vi "Init.vi"(8 "error in (no error)":errorcluster, 11 "DataTable in":refnum<class "DataTable.lvclass">) -> (0 "error out":errorcluster, 3 "DataTable out":refnum<class "DataTable.lvclass">)   [LabVIEW 2016, in "DataGrid.lvlib" / "DataTable.lvclass"]
doc: ".NET datatable constructor, puts the .net reference into the class"
uses:
  <userlib>/LabVIEWdotNetDataGrid/source/DataTable/DataTable.lvclass
  System.Data
  <userlib>/LabVIEWdotNetDataGrid/source/DataTable/DataTable.lvclass/DataTable.ctl
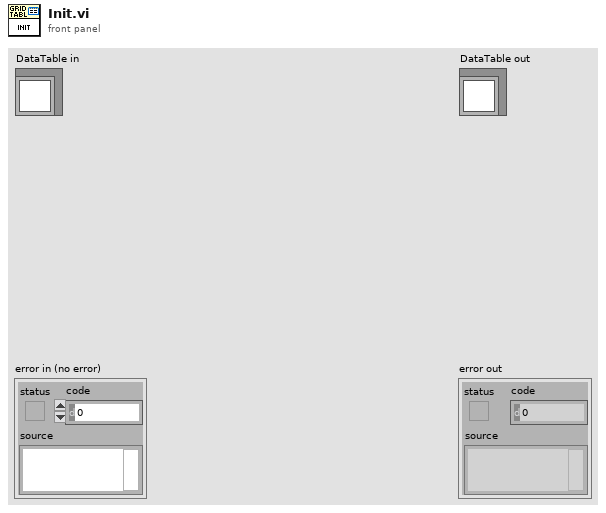
[diagram p1: front panel]
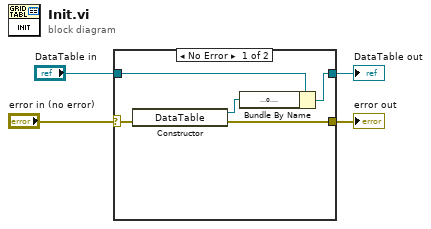
[diagram p0: block diagram]
diagram:
  n1 = case shown="No Error" "error in (no error)" {
    selector: "error in (no error)" -> [w8 w11]
    tunnel: [w5 w11] -> w3
    tunnel: [w6 w10] -> w1
    tunnel: "DataTable in" -> [w7 w10]
    frame No Error {
      n2 = constructor class="DataTable"(error in=w8) -> (reference out=w9:refnum<k24>, error out=w5:errorcluster)  [unwired: 2 in, 1 out]
      n3 = Bundle By Name(cluster=w7, "DataTable"=w9) -> (w6:refnum<class "DataTable.lvclass">)
    }
    frame Error {
    }
  }
  "error out" <- w3
  "DataTable out" <- w1
